vi "FTW-DevUtil-ActorsInMemory.vi"() -> ()   [LabVIEW 2013]
uses:
  <vilib>/Utility/VariantDataType/VariantType.lvlib
  source/actor/Instance/FTW-ActorInstance.lvclass
panel:
  out "Update Time":dbl format="%.3f sec"
  in  "Active Actors":i32(listbox)
  # "Double click to open FP. Ctrl+Double Click to open BD."
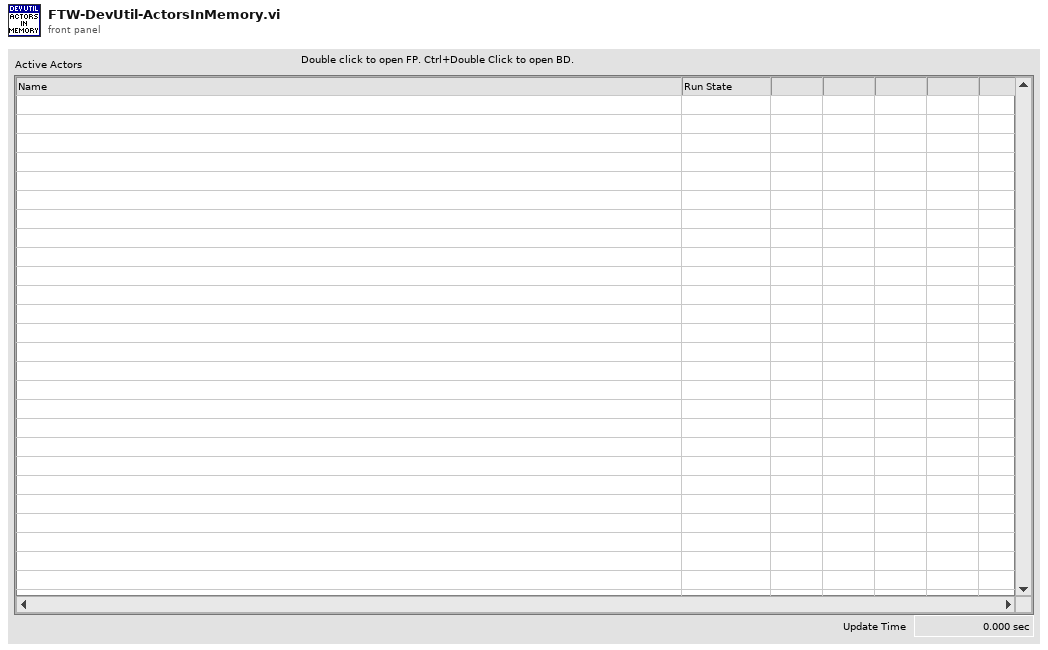
[diagram p1: front panel]
types:
  T1 = typedef "VariantType.lvlib/Type.ctl" = enum8{"Invalid Type", "Void", "I8", "I16", "I32", "I64", "U8", "U16", "U32", "U64", "Single Float", "Double Float", "Extended Float", "Single Complex", "Double Complex", "Extended Complex", "Enum U8", "Enum U16", "Enum U32", "Enum U64", "Single Float With Unit", "Double Float With Unit", "Extended Float With Unit", "Single Complex with Unit", "Double Complex with Unit", "Extended Complex with Unit", "Boolean", "String", "Path", "Picture", "Tag", "Array", "Cluster", "Variant", "LV Variant", "Waveform", "Timestamp", "Digital Waveform", "Digital Data", "ExpressData", "Refnum", "External Data", "VI", "Poly VI", "LabVIEW Class Instance", "Fixed Point"}
  T2 = enum32{"Bad", "Idle", "Run top level", "Running"}
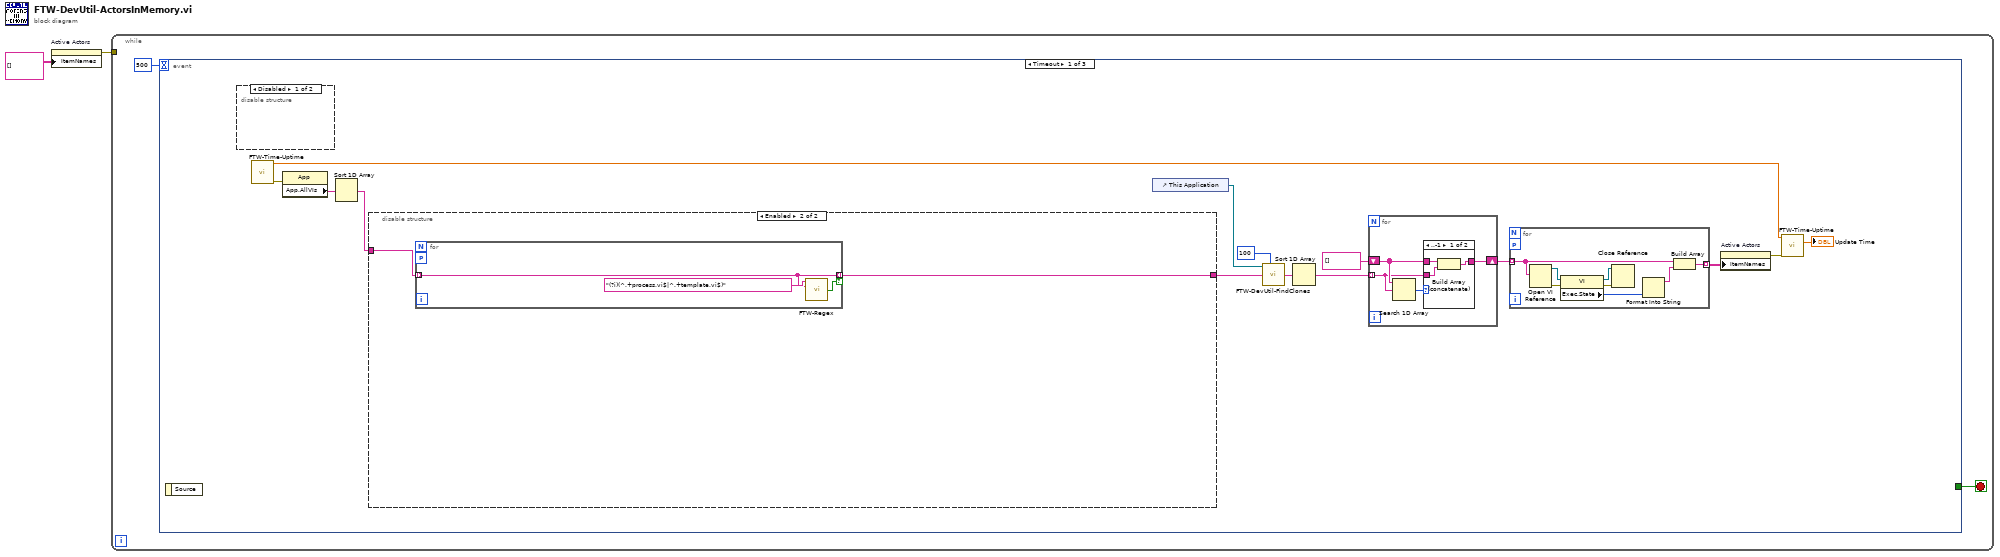
[diagram p0: block diagram]
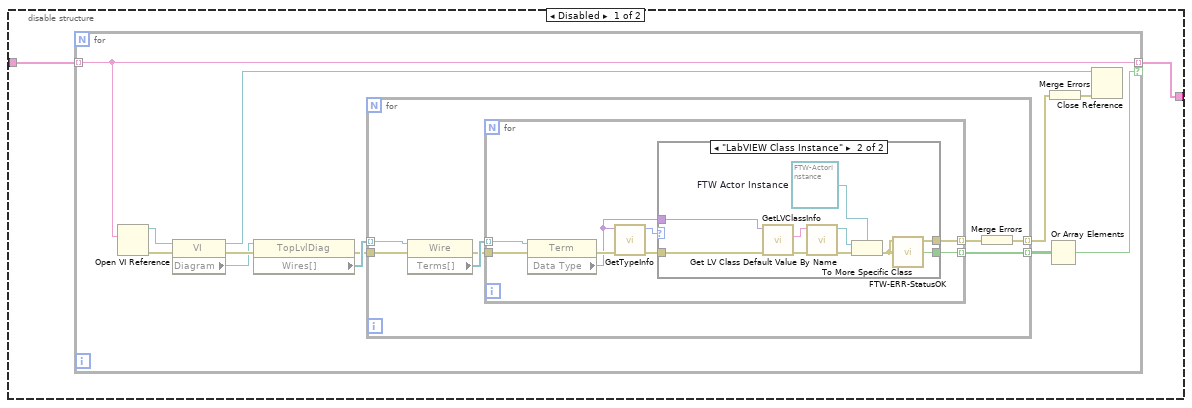
[diagram p3: hidden frame]
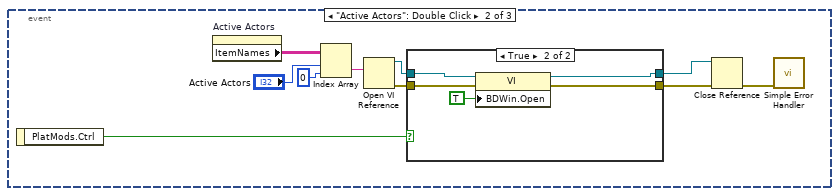
[diagram p6: hidden frame]
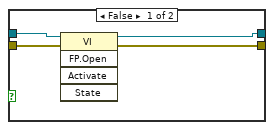
[diagram p7: hidden frame]
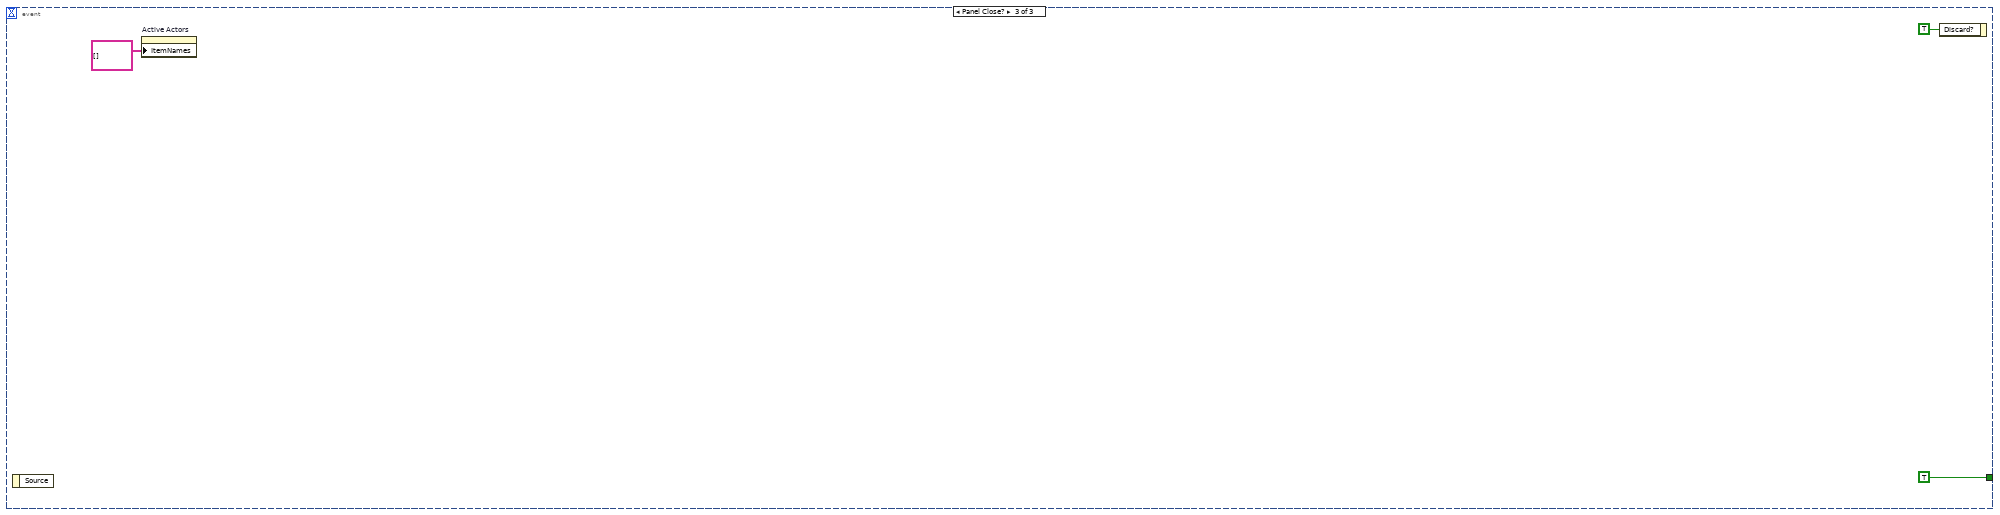
[diagram p8: hidden frame]
diagram:
  n1 = property on="Active Actors" class="MCListbox (strict)"("ItemNames"=string[][] [] ("Item Names")) -> (error out=w1:errorcluster)  [unwired: 2 in, 1 out]
  n2 = while {
    tunnel: w1 -> [_]
    stop <- w3 stop-if-true
    n3 = event shown="[0] Timeout" {
      selector: _ -> [_ _ _]
      dyn-events: _ -> [_ _ _]
      timeout: 500 -> [_ _ _]
      tunnel: [_ _ TRUE] -> w3
      event Timeout {
        n4 = event-data() -> ()  [unwired: 1 in, 1 out]
        n5 = disable-structure shown="Disabled" {
          frame Disabled {
          }
          frame Enabled {
          }
        }
        n6 = call "FTW-Time-Uptime.vi"() -> ("Current Uptime"=w6:dbl, "error out"=w7:errorcluster)  [unwired: 13 in, 1 out]
        n7 = property class="App"(error in=w7) -> ("App.AllVIs"=w15:string[])  [unwired: 1 in, 2 out]
        n8 = Sort 1D Array(array=w15) -> (sorted array=w18:string[])
        n9 = disable-structure shown="Enabled" {
          disable-tunnel: w18 -> [w28 w67]
          disable-tunnel: [w27 w66] -> w14
          frame Disabled {
            n10 = for {
              tunnel: w28 -> [w36] mode=indexing
              tunnel: [w36] -> w27 mode=indexing if=w32
              n11 = Open VI Reference(vi path=w36) -> (vi reference=w40:refnum<vi>, error out=w39:errorcluster)  [unwired: 5 in]
              n12 = property class="VI"(reference=w40, error in=w39) -> (reference out=w37:refnum<vi>, error out=w38:errorcluster, "Diagram"=w35:refnum<vi>)
              n13 = property class="TopLvlDiag"(reference=w35, error in=w38) -> (error out=w31:errorcluster, "Wires[]"=w34:refnum<vi>[])  [unwired: 1 out]
              n14 = for {
                tunnel: w34 -> [w47] mode=indexing
                tunnel: [w44] -> w33 mode=indexing
                tunnel: w31 -> [w43]
                tunnel: [w41] -> w30 mode=indexing
                n15 = property class="Wire"(reference=w47, error in=w43) -> (error out=w45:errorcluster, "Terms[]"=w46:refnum<vi>[])  [unwired: 1 out]
                n16 = for {
                  tunnel: w46 -> [w55] mode=indexing
                  tunnel: w45 -> [w54]
                  tunnel: [w49] -> w44 mode=indexing
                  tunnel: [w48] -> w42 mode=indexing
                  n17 = property class="Term"(reference=w55, error in=w54) -> (error out=w53:errorcluster, "Data Type"=w51:variant)  [unwired: 1 out]
                  n18 = call <vilib>:"GetTypeInfo.vi"("error in (no error)"=w53, "Variant"=w51) -> ("error out"=w50:errorcluster, "Type Enum"=w52:T1)  [unwired: 5 in, 3 out]
                  n19 = case shown="\"LabVIEW Class Instance\"" w52 {
                    tunnel: w51 -> [_ w65]
                    tunnel: w50 -> [w56 w64]
                    tunnel: [_ w59] -> w49
                    tunnel: [w56 w58] -> w48
                    frame "Invalid Type", Default {
                    }
                    frame "LabVIEW Class Instance" {
                      w57 = refnum<class "FTW-ActorInstance.lvclass"> refnum  # FTW Actor Instance
                      n20 = call <vilib>:"GetLVClassInfo.vi"("error in (no error)"=w64, "Variant"=w65) -> ("error out"=w62:errorcluster, "LV Class File Name"=w63:string)  [unwired: 7 in, 1 out]
                      n21 = call <vilib>:"Get LV Class Default Value By Name.vi"("error in (no error)"=w62, "class name"=w63) -> ("error out"=w61:errorcluster, "object"=w60:refnum<class>)  [unwired: 8 in]
                      n22 = To More Specific Class(target class=w57, reference=w60, error in=w61) -> (error out=w58:errorcluster)  [unwired: 1 out]
                      n23 = call "FTW-ERR-StatusOK.vi"("error to check"=w58) -> ("Status OK?"=w59:bool)
                    }
                  }
                }
                n24 = Merge Errors(w42) -> (w41:errorcluster)
              }
              n25 = Or Array Elements(Boolean array=w33) -> (logical OR=w32:bool)
              n26 = Merge Errors(w30) -> (w29:errorcluster)
              n27 = Close Reference(reference=w37, error in (no error)=w29) -> ()  [unwired: 1 out]
            }
          }
          frame Enabled {
            n28 = for {
              tunnel: w67 -> [w69] mode=indexing
              tunnel: [w69] -> w66 mode=indexing if=w68
              workers-P: _ -> [_]
              n29 = call "FTW-Regex.vi"("Regular Expression"="(?i)(^.+process.vi$|^.+template.vi$)", "Input String"=w69) -> ("Match Found?"=w68:bool)  [unwired: 9 in, 4 out]
            }
          }
        }
        n30 = control-ref of="This Application"() -> (w17:refnum<vi>)
        n31 = call "FTW-DevUtil-FindClones.vi"("Application in"=w17, "Search Clones Up To"=100, "VIs in"=w14) -> ("VIs (including clones) out"=w13:string[])  [unwired: 12 in]
        n32 = Sort 1D Array(array=w13) -> (sorted array=w11:string[])
        n33 = for {
          tunnel: w11 -> [w19] mode=indexing
          shift-right: [w21] -> w9
          shift-left: string[] [] -> [w20]
          n34 = Search 1D Array(1D array=w20, element=w19) -> (index of element=w22:i32)  [unwired: 1 in]
          n35 = case shown="..-1" w22 {
            tunnel: [w24 w26] -> w21
            tunnel: w20 -> [w25 w26]
            tunnel: w19 -> [w23 _]
            frame ..-1 {
              n36 = Build Array (concatenate)(w25, w23) -> (w24:string[])
            }
            frame 0.. {
            }
          }
        }
        n37 = for {
          tunnel: w9 -> [w74] mode=indexing
          tunnel: [w72] -> w12 mode=indexing
          workers-P: _ -> [_]
          n38 = Open VI Reference(vi path=w74) -> (vi reference=w78:refnum<vi>, error out=w77:errorcluster)  [unwired: 5 in]
          n39 = property class="VI"(reference=w78, error in=w77) -> (reference out=w76:refnum<vi>, error out=w71:errorcluster, "Exec.State"=w75:T2)
          n40 = Close Reference(reference=w76, error in (no error)=w71) -> ()  [unwired: 1 out]
          n41 = Format Into String(w75) -> (resulting string=w73:string)  [unwired: 3 in, 1 out]
          n42 = Build Array(w74, w73) -> (w72:string[])
        }
        n43 = property on="Active Actors" class="MCListbox (strict)"("ItemNames"=w12) -> (error out=w8:errorcluster)  [unwired: 2 in, 1 out]
        n44 = call "FTW-Time-Uptime.vi"("Previous Uptime"=w6, "error in"=w8) -> ("Elapsed Time"=→"Update Time":dbl)  [unwired: 11 in, 2 out]
      }
      event "Active Actors": Double Click {
        n45 = event-data() -> ("PlatMods.Ctrl"=w79:bool)  [unwired: 1 in]
        n46 = property on="Active Actors" class="MCListbox (strict)"() -> ("ItemNames"=w88:string[][])  [unwired: 2 in, 2 out]
        n47 = Index Array(array=w88, index (row)="Active Actors", index (col)=0 ("disabled index (col)")) -> (element=w85:string)
        n48 = Open VI Reference(vi path=w85) -> (vi reference=w84:refnum<vi>, error out=w83:errorcluster)  [unwired: 5 in]
        n49 = case shown="True" w79 {
          tunnel: w84 -> [w92 w95]
          tunnel: w83 -> [w91 w97]
          tunnel: [w90 w96] -> w82
          tunnel: [w89 w94] -> w81
          frame False {
            n50 = invoke class="VI" method="FP.Open"(reference=w92, error in=w91) -> (reference out=w89:refnum<vi>, error out=w90:errorcluster)  [unwired: 3 in, 3 out]
          }
          frame True {
            n51 = property class="VI"(reference=w95, error in=w97, "BDWin.Open"=TRUE ("Block Diagram Window:Open")) -> (reference out=w94:refnum<vi>, error out=w96:errorcluster)
          }
        }
        n52 = Close Reference(reference=w81, error in (no error)=w82) -> (error out=w80:errorcluster)
        n53 = call <vilib>:"Simple Error Handler.vi"("error in (no error)"=w80) -> ()  [unwired: 4 in, 5 out]
      }
      event Panel Close? {
        n54 = event-data() -> ()  [unwired: 1 in, 1 out]
        n55 = property on="Active Actors" class="MCListbox (strict)"("ItemNames"=string[][] [] ("Item Names")) -> ()  [unwired: 2 in, 2 out]
        n56 = event-data("Discard?"=TRUE) -> ()  [unwired: 1 in, 1 out]
      }
    }
  }
